vi "Hierarchical VArray to MultiD Array.vi"(8 "error in (no error)":errorcluster, 10 "Hierarchical Array":variant[](array[variant])) -> (0 "error out":errorcluster, 2 "MultiD Array":variant)   [LabVIEW 2013, in "JKI JSON Serialization.lvlib" / "JSON Deserializer.lvclass"]
uses:
  JSON Deserializer.lvclass
  <vilib>/Utility/VariantDataType/VariantType.lvlib
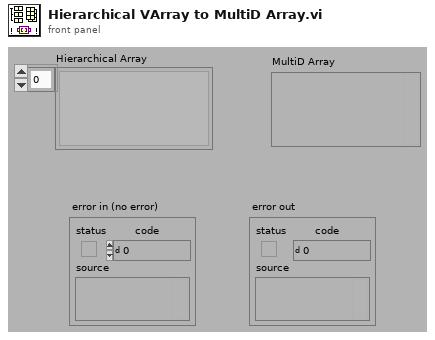
[diagram p1: front panel]
types:
  T1 = typedef "VariantType.lvlib/Type.ctl" = enum8{"Invalid Type", "Void", "I8", "I16", "I32", "I64", "U8", "U16", "U32", "U64", "Single Float", "Double Float", "Extended Float", "Single Complex", "Double Complex", "Extended Complex", "Enum U8", "Enum U16", "Enum U32", "Enum U64", "Single Float With Unit", "Double Float With Unit", "Extended Float With Unit", "Single Complex with Unit", "Double Complex with Unit", "Extended Complex with Unit", "Boolean", "String", "Path", "Picture", "Tag", "Array", "Cluster", "Variant", "LV Variant", "Waveform", "Timestamp", "Digital Waveform", "Digital Data", "ExpressData", "Refnum", "External Data", "VI", "Poly VI", "LabVIEW Class Instance", "Fixed Point"}
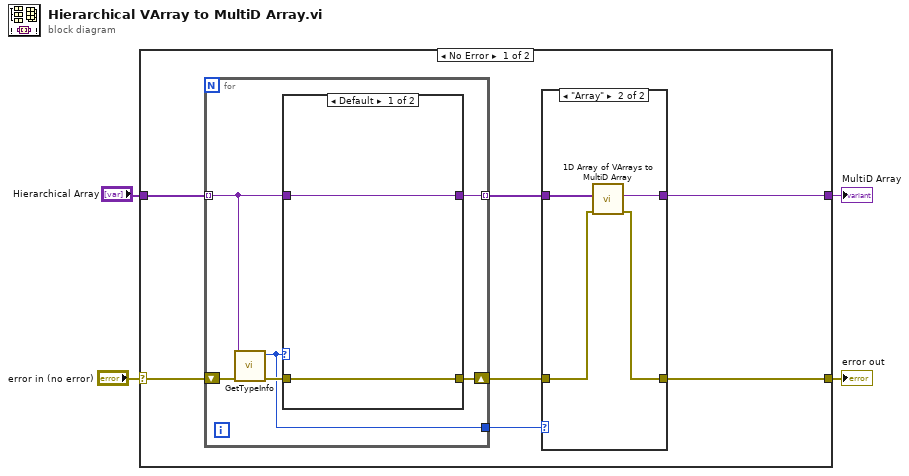
[diagram p0: block diagram]
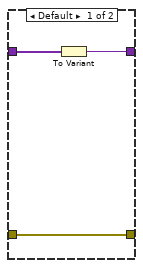
[diagram p2: hidden frame]
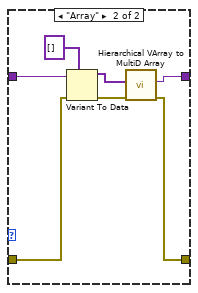
[diagram p3: hidden frame]
diagram:
  n1 = case shown="No Error" "error in (no error)" {
    selector: "error in (no error)" -> [w10 w34]
    tunnel: [w7 w34] -> w4
    tunnel: [w6 _] -> w1
    tunnel: "Hierarchical Array" -> [w11 _]
    frame No Error {
      n2 = for {
        tunnel: w11 -> [w21] mode=indexing
        shift-right: [w23] -> w8
        shift-left: w10 -> [w24]
        tunnel: [w20] -> w9 mode=indexing
        tunnel: [w19] -> w5
        n3 = call <vilib>:"GetTypeInfo.vi"("error in (no error)"=w24, "Variant"=w21) -> ("error out"=w22:errorcluster, "Type Enum"=w19:T1)  [unwired: 5 in, 3 out]
        n4 = case shown="Default" w19 {
          tunnel: [w25 w28] -> w23
          tunnel: w22 -> [w25 w27]
          tunnel: w21 -> [w26 w33]
          tunnel: [w26 w29] -> w20
          frame Default {
          }
          frame "Array" {
            n5 = Variant To Data(error in=w27, type=variant[] [], Variant=w33) -> (data=w31:variant[], error out=w30:errorcluster)
            n6 = call "Hierarchical VArray to MultiD Array.vi"("error in (no error)"=w30, "Hierarchical Array"=w31) -> ("error out"=w28:errorcluster, "MultiD Array"=w29:variant)  [unwired: 8 in]
          }
        }
      }
      n7 = case shown="\"Array\"" w5 {
        tunnel: w9 -> [w13 w18]
        tunnel: w8 -> [w12 w17]
        tunnel: [w12 w16] -> w7
        tunnel: [w14 w15] -> w6
        frame Default {
          n8 = To Variant(anything=w13) -> (Variant=w14:variant)
        }
        frame "Array" {
          n9 = call "1D Array of VArrays to MultiD Array.vi"("error in (no error)"=w17, "Array of VArrays"=w18) -> ("error out"=w16:errorcluster, "MultiD Array"=w15:variant)  [unwired: 8 in]
        }
      }
    }
    frame Error {
    }
  }
  "error out" <- w4
  "MultiD Array" <- w1
